vi "Main.vi"() -> ()   [LabVIEW 2016]
doc: "This template is for the Queued Message Handler design pattern.\n\nThe Event Handling Loop generates messages based on user interface actions.\n\nThe Message Handling Loop processes messages generated by the Event Handling Loop, or by other messages. The messages are string values, so new messages can be added easily to the Message Cases case structure in the Message Handling Loop. Each message cluster can also provide an optional value for Message Data, which is a variant that can be converted to whatever message-specific data is required."
uses:
  controls/UI Data.ctl
  controls/Model_Controller Data.ctl
  controls/LV Version Details.ctl
  support/Message Queue/Enqueue Message (Single).vi
  <vilib>/xml/Load XML File.vi
  <vilib>/Utility/error.llb/Error Cluster From Error Code.vi
  <vilib>/ErrorRing/Error Ring.xnode
  support/Message Queue/Message Queue.lvlib
  support/User Event - Stop/User Event - Stop.lvlib
  <vilib>/xml/NI_XML.lvlib
panel:
  in  "OpenInLV":bool
  in  "LV Version":u16(ring) caption="LabVIEW Version" items=["LabVIEW 2014 SP1 32-bit", "LabVIEW 2016 32-bit", "LabVIEW 2017 SP1 32-bit", "LabVIEW 2019 SP1 f1 32-bit"]
  out "Load Time (ms)":u32
  out "DS":T1(array[cluster])
  out "parse errors":string
  in  "LV Project Viewer":string(tree)
  in  "LVProject File Path":path
  in  "Do Something Else <Replace Me>":bool
  in  "Do Something <Replace Me>":bool
  in  "Exit":bool
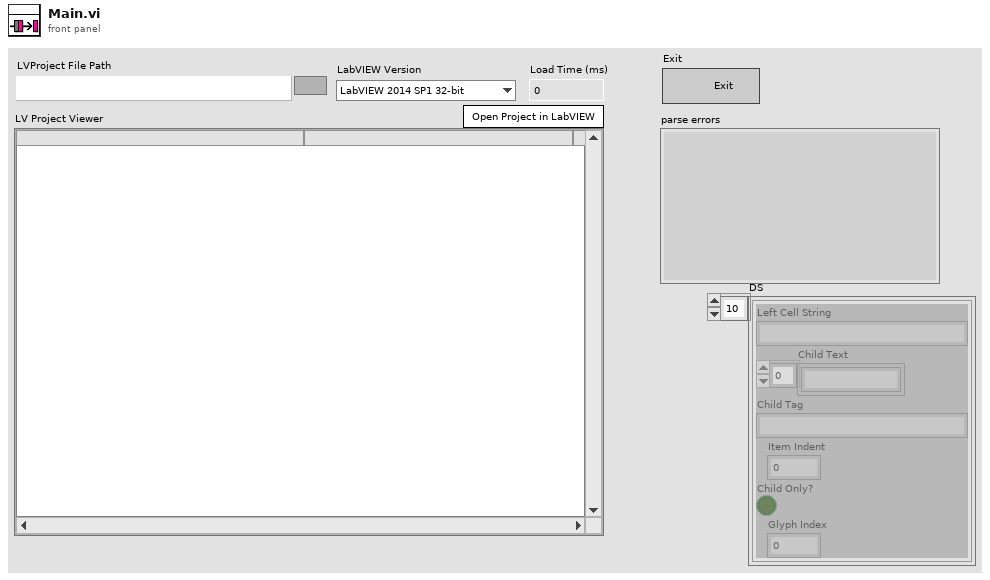
[diagram p1: front panel]
types:
  T1 = cluster{"Left Cell String":string, "Child Text":string[], "Child Tag":string, "Item Indent":i32, "Child Only?":bool, "Glyph Index":i32}[]
  T2 = typedef "Model_Controller Data.ctl" = cluster{"LVProj XML String":string, "LV Proj XML DOM":refnum<k20>, "DS":cluster{"Left Cell String":string, "Child Text":string[], "Child Tag":string, "Item Indent":i32, "Child Only?":bool, "Glyph Index":i32}[], "LV Version Details":T3[], "Selected LV Version":T3, "Item to open in LV":string}
  T3 = typedef "LV Version Details.ctl" = cluster{"Bitness":string, "Version String":string, "LV EXE Path":path, "Display Name":string, "Version":string}
  T4 = typedef "UI Data.ctl" = cluster{"Exit Button Ref":refnum<vi>, "LV Proj File Path":path, "LV Proj View Tree":refnum<vi>}
  T5 = typedef "Message Queue.lvlib/All Message Queues.ctl" = cluster{"UI":refnum<queue>}
  T6 = typedef "imagedata.ctl" = cluster{"image type":i32, "image depth":i32, "image":u8[], "mask":u8[], "colors":u32[], "Rectangle":cluster{"left":i16, "top":i16, "right":i16, "bottom":i16}}
  T7 = cluster{"Left Cell String":string, "Child Text":string[], "Child Tag":string, "Item Indent":i32, "Child Only?":bool, "Glyph Index":i32}
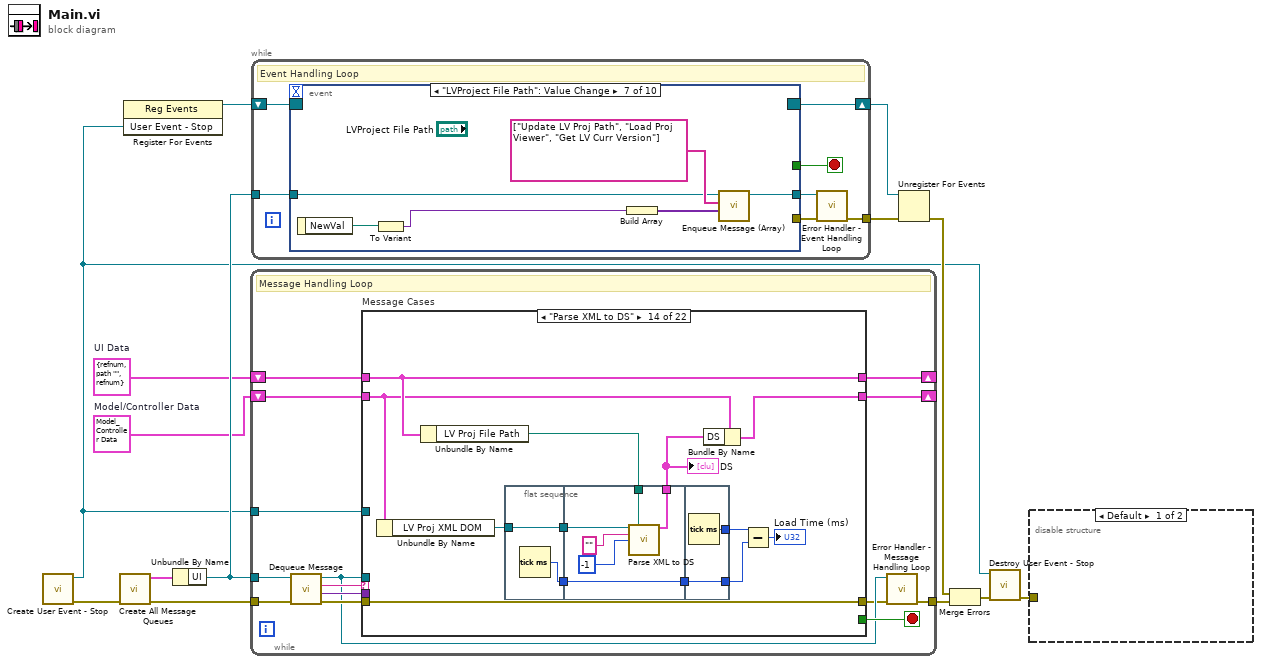
[diagram p0: block diagram]
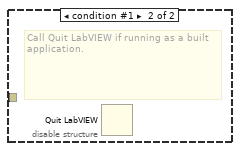
[diagram p2: hidden frame]
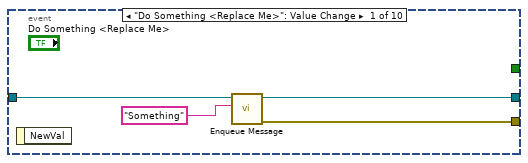
[diagram p3: hidden frame]
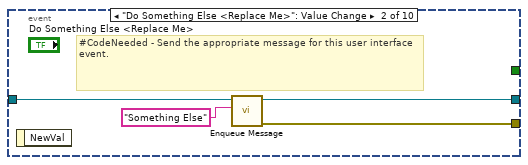
[diagram p4: hidden frame]
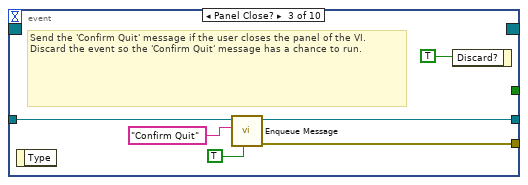
[diagram p5: hidden frame]
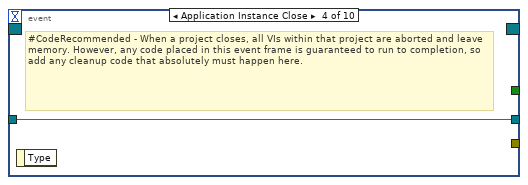
[diagram p6: hidden frame]
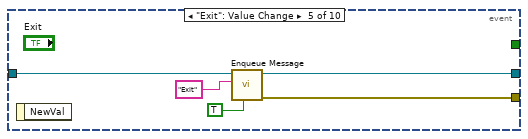
[diagram p7: hidden frame]
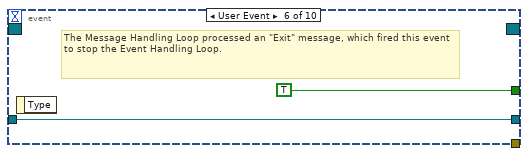
[diagram p8: hidden frame]
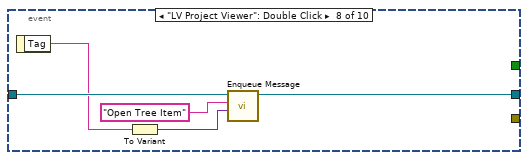
[diagram p9: hidden frame]
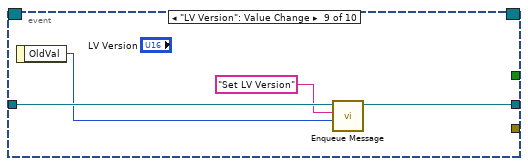
[diagram p10: hidden frame]
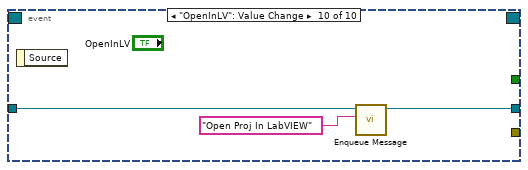
[diagram p11: hidden frame]
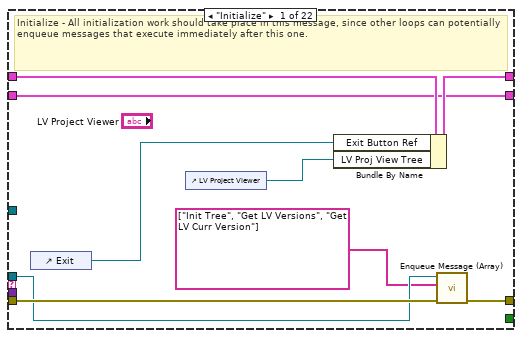
[diagram p12: hidden frame]
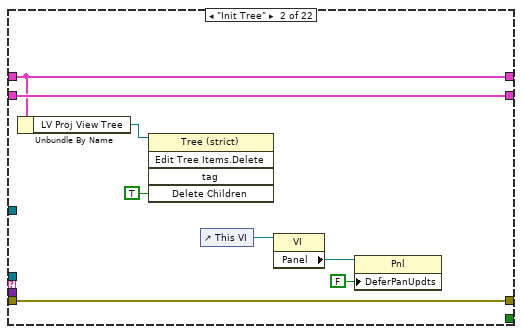
[diagram p13: hidden frame]
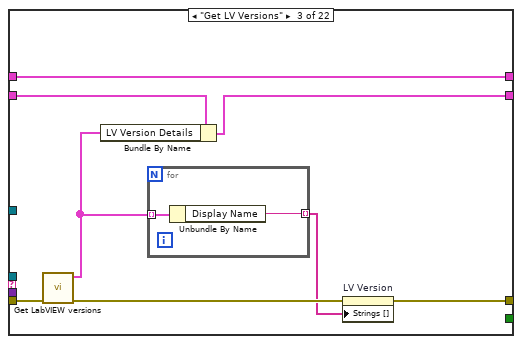
[diagram p14: hidden frame]
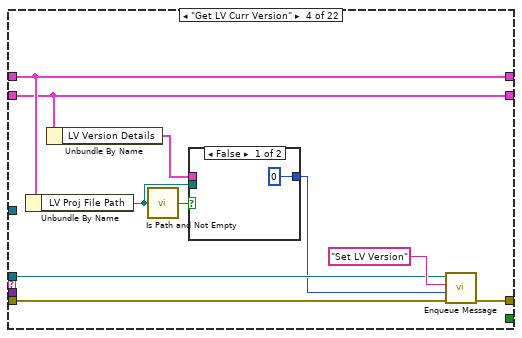
[diagram p15: hidden frame]
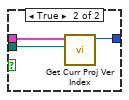
[diagram p16: hidden frame]
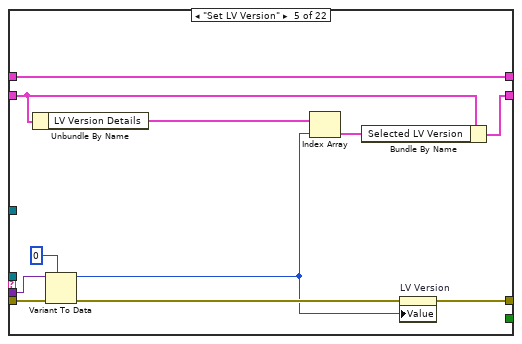
[diagram p17: hidden frame]
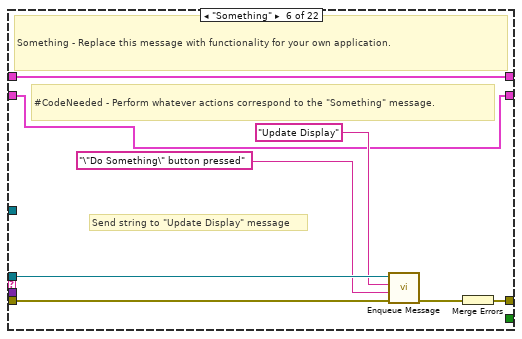
[diagram p18: hidden frame]
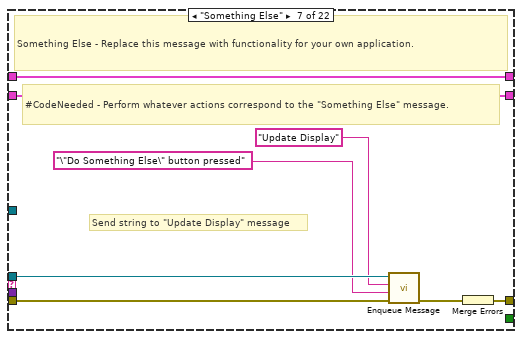
[diagram p19: hidden frame]
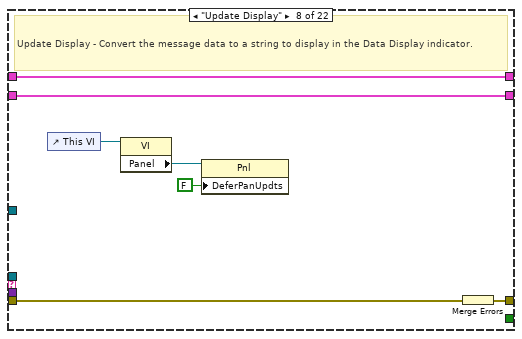
[diagram p20: hidden frame]
diagram:
  w1 = T2 {"LVProj XML String"="", "LV Proj XML DOM"=refnum, "DS"=[], "LV Version Details"=[], "Selected LV Version"={"Bitness"="", "Version String"="", "LV EXE Path"=path "", "Display Name"="", "Version"=""}, "Item to open in LV"=""}  # Model/Controller Data
  w6 = T4 {"Exit Button Ref"=refnum, "LV Proj File Path"=path "", "LV Proj View Tree"=refnum}  # UI Data
  n1 = call "Create User Event - Stop.vi"() -> ("error out"=w10:errorcluster, "User Event - Stop"=w2:refnum<user-event>)  [unwired: 10 in]
  n2 = call "Create All Message Queues.vi"("error in (no error)"=w10) -> ("error out"=w14:errorcluster, "Message Queues out"=w13:T5)  [unwired: 9 in]
  n3 = register-events(w2) -> (reference out=w3:refnum<event-registration>)  [unwired: 2 in, 1 out]
  n4 = Unbundle By Name(w13) -> ("UI"=w11:refnum<queue>)
  n5 = while {
    tunnel: w11 -> [w20]
    shift-right: [w27] -> _
    shift-left: w6 -> [w28]
    tunnel: w2 -> [w25]
    tunnel: w14 -> [w24]
    tunnel: [w18] -> w12
    shift-right: [w15] -> _
    shift-left: w1 -> [w16]
    stop <- w26 stop-if-true
    # "Message Handling Loop"
    n6 = call "Dequeue Message.vi"("error in (no error)"=w24, "Message Queue"=w20) -> ("error out"=w23:errorcluster, "Message Data"=w21:variant, "Message"=w22:string, "dup Message Queue"=w19:refnum<queue>)  [unwired: 6 in]
    n7 = case "Message Cases" shown="\"Parse XML to DS\"" w22 {
      selector: w22 -> [_ _ _ _ _ _ _ _ _ _ _ _ _ _ _ _ _ _ _ _ _ w242]
      tunnel: w19 -> [w30 _ _ w57 _ w84 w92 _ _ w115 w121 _ _ _ _ _ _ w194 w215 _ w240 _]
      tunnel: w23 -> [w32 w45 w52 w59 w79 w86 w94 w101 w111 w119 w123 w133 w142 w156 w172 w183 w190 w205 w217 w224 w233 _]
      tunnel: [w31 w45 w48 w58 w73 w87 w95 w102 w105 w117 w125 w135 w141 w156 w172 w183 w190 w195 w216 w223 w236 w243] -> w17
      tunnel: w28 -> [w37 w42 w53 w63 w80 w88 w96 w103 w110 w118 w126 w128 w143 w154 w170 w178 w189 w200 w218 w222 w239 w244]
      tunnel: [w36 w42 w53 w63 w80 w88 w96 w103 w110 w118 w126 w127 w143 w154 w170 w178 w189 w200 w218 w222 w239 w244] -> w27
      tunnel: [_ _ _ _ _ _ _ _ _ _ _ _ _ _ _ _ _ _ _ _ TRUE _] -> w26
      tunnel: w21 -> [_ _ _ _ w78 _ _ _ w109 _ _ w131 _ _ _ _ _ w204 _ _ w230 _]
      tunnel: w25 -> [_ _ _ _ _ _ _ _ _ _ _ _ _ _ _ _ _ _ _ _ w235 _]
      tunnel: w16 -> [w34 w44 w51 w61 w71 w81 w89 w100 w104 w112 w124 w134 w138 w152 w171 w176 w188 w193 w213 w221 w229 w241]
      tunnel: [w34 w44 w50 w61 w70 w81 w89 w100 w104 w112 w124 w134 w137 w151 w171 w176 w188 w192 w212 w221 w229 w241] -> w15
      frame "Initialize" {
        # "Initialize - All initialization work should take place in this message, since other loops can potentially enqueue messages that execute immediately after this one."
        n8 = control-ref of="Exit"() -> (w35:refnum<vi>)
        n9 = control-ref of="LV Project Viewer"() -> (w33:refnum<vi>)
        n10 = Bundle By Name(cluster=w37, "Exit Button Ref"=w35, "LV Proj View Tree"=w33) -> (w36:T4)
        n11 = call "Enqueue Message (Array).vi"("error in (no error)"=w32, "Message Array"=string[] ["Init Tree", "Get LV Versions", "Get LV Curr Version"], "Message Queue"=w30) -> ("error out"=w31:errorcluster)  [unwired: 7 in, 1 out]
      }
      frame "Init Tree" {
        n12 = Unbundle By Name(w42) -> ("LV Proj View Tree"=w41:refnum<vi>)
        n13 = invoke class="Tree (strict)" method="Edit Tree Items.Delete"(reference=w41, "Delete Children"=TRUE ("Delete Children?")) -> ()  [unwired: 3 in, 5 out]
        n14 = control-ref of="This VI"() -> (w40:refnum<vi>)
        n15 = property class="VI"(reference=w40) -> ("Panel"=w39:refnum<vi>)  [unwired: 1 in, 2 out]
        n16 = property class="Pnl"(reference=w39, "DeferPanUpdts"=FALSE ("Defer Panel Updates")) -> ()  [unwired: 1 in, 2 out]
      }
      frame "Get LV Versions" {
        n17 = call "Get LabVIEW versions.vi"("error in (no error)"=w52) -> ("error out"=w49:errorcluster, "LV Version Details"=w47:T3[])  [unwired: 9 in]
        n18 = Bundle By Name(cluster=w51, "LV Version Details"=w47) -> (w50:T2)
        n19 = for {
          tunnel: w47 -> [w55] mode=indexing
          tunnel: [w54] -> w46 mode=indexing
          n20 = Unbundle By Name(w55) -> ("Display Name"=w54:string)
        }
        n21 = property on="LV Version" class="Ring (strict)"(error in=w49, "Strings []"=w46) -> (error out=w48:errorcluster)  [unwired: 1 in, 1 out]
      }
      frame "Get LV Curr Version" {
        n22 = Unbundle By Name(w63) -> ("LV Proj File Path"=w65:path)
        n23 = Unbundle By Name(w61) -> ("LV Version Details"=w62:T3[])
        n24 = call <vilib>:"Is Path and Not Empty.vi"("path"=w65) -> ("Is Path and Not Empty?"=w64:bool)  [unwired: 4 in]
        n25 = case shown="False" w64 {
          tunnel: w65 -> [_ w69]
          tunnel: w62 -> [_ w68]
          tunnel: [0 ("Proj LV Ver Index") w67] -> w56
          frame False {
          }
          frame True {
            n26 = call "Get Curr Proj Ver Index.vi"("LV Proj File Path"=w69, "LV Version Details"=w68) -> ("Proj LV Ver Index"=w67:i32)  [unwired: 9 in]
          }
        }
        n27 = call-poly "Enqueue Message.vi"("error in (no error)"=w59, "Message Data"=w56, "Message"="Set LV Version", "Message Queue"=w57) -> ("error out"=w58:errorcluster)  [unwired: 6 in, 1 out]
      }
      frame "Set LV Version" {
        n28 = Unbundle By Name(w71) -> ("LV Version Details"=w75:T3[])
        n29 = Variant To Data(error in=w79, type=u16 0, Variant=w78) -> (data=w72:u16, error out=w74:errorcluster)
        n30 = Index Array(array=w75, index=w72) -> (element=w76:T3)
        n31 = Bundle By Name(cluster=w71, "Selected LV Version"=w76) -> (w70:T2)
        n32 = property on="LV Version" class="Ring (strict)"(error in=w74, "Value"=w72) -> (error out=w73:errorcluster)  [unwired: 1 in, 1 out]
      }
      frame "Something" {
        # "Send string to \"Update Display\" message"
        # "#CodeNeeded - Perform whatever actions correspond to the \"Something\" message."
        # "Something - Replace this message with functionality for your own application."
        n33 = call-poly "Enqueue Message.vi"("error in (no error)"=w86, "Message Data"="\"Do Something\" button pressed" ("\"Do Something\" button pressed"), "Message"="Update Display", "Message Queue"=w84) -> ("error out"=w85:errorcluster)  [unwired: 6 in, 1 out]
        n34 = Merge Errors(w85) -> (w87:errorcluster)
      }
      frame "Something Else" {
        # "Send string to \"Update Display\" message"
        # "#CodeNeeded - Perform whatever actions correspond to the \"Something Else\" message."
        # "Something Else - Replace this message with functionality for your own application."
        n35 = call-poly "Enqueue Message.vi"("error in (no error)"=w94, "Message Data"="\"Do Something Else\" button pressed" ("\"Do Something Else\" button pressed"), "Message"="Update Display", "Message Queue"=w92) -> ("error out"=w93:errorcluster)  [unwired: 6 in, 1 out]
        n36 = Merge Errors(w93) -> (w95:errorcluster)
      }
      frame "Update Display" {
        # "Update Display - Convert the message data to a string to display in the Data Display indicator."
        n37 = control-ref of="This VI"() -> (w99:refnum<vi>)
        n38 = property class="VI"(reference=w99) -> ("Panel"=w98:refnum<vi>)  [unwired: 1 in, 2 out]
        n39 = property class="Pnl"(reference=w98, "DeferPanUpdts"=FALSE ("Defer Panel Updates")) -> ()  [unwired: 1 in, 2 out]
        n40 = Merge Errors(w101) -> (w102:errorcluster)
      }
      frame "Error" {
        # "#CodeRecommended - If you ever change the name of this \"Error\" message, you'll need to update the name in the Check Loop Error.vi as well."
        # "#CodeRecommended - Consider creating a system for logging errors in some way. These errors are for notification purposes only. Handling of specific errors should be performed in the message frames that generated the error."
        # "Error - Display an error dialog. This message is sent by the \"Error Handler\" VIs at the end of other loops in this application."
        n41 = Variant To Data(error in=w111, type=errorcluster {"status"=FALSE, "code"=0, "source"=""} ("error constant"), Variant=w109) -> (data=w107:errorcluster, error out=w106:errorcluster)
        n42 = call <vilib>:"Simple Error Handler.vi"("error in (no error)"=w107) -> ()  [unwired: 4 in, 5 out]
        n43 = Merge Errors(w106) -> (w105:errorcluster)
      }
      frame "Confirm Quit" {
        # "#CodeNeeded - If you want to provide an \"Are you sure\" dialog (or some other notification) before the application exits, place that code here. This message is typically sent from a Panel Close? event."
        # "Confirm Quit - Message that can confirm whether or not the user wants to exit the application."
        n44 = call-poly "Enqueue Message.vi"("Priority Message? (F)"=TRUE, "error in (no error)"=w119, "Message"="Exit", "Message Queue"=w115) -> ("error out"=w116:errorcluster)  [unwired: 6 in, 1 out]
        n45 = Merge Errors(w116) -> (w117:errorcluster)
      }
      frame "Load Proj Viewer" {
        n46 = call "Enqueue Message (Array).vi"("error in (no error)"=w123, "Message Array"=string[] ["Init Tree", "Read Proj XML", "Parse XML to DS", "Add Custom Symbols", "Populate Nodes", "Close All", "Update Display"], "Message Queue"=w121) -> ("error out"=w122:errorcluster)  [unwired: 7 in, 1 out]
        n47 = Merge Errors(w122) -> (w125:errorcluster)
      }
      frame "Update LV Proj Path" {
        n48 = Variant To Data(error in=w133, type=path "", Variant=w131) -> (data=w129:path, error out=w132:errorcluster)
        n49 = Bundle By Name(cluster=w128, "LV Proj File Path"=w129) -> (w127:T4)
        n50 = Merge Errors(w132) -> (w135:errorcluster)
      }
      frame "Read Proj XML" {
        n51 = Unbundle By Name(w143) -> ("LV Proj File Path"=w140:path)
        n52 = call-poly <vilib>:"Load.vi"("path to XML document"=w140, "error in (no error)"=w142) -> ("DOM document out"=w139:refnum<k20>, "parse errors"=→"parse errors":string, "error out"=w141:errorcluster)  [unwired: 11 in]
        n53 = Bundle By Name(cluster=w138, "LV Proj XML DOM"=w139) -> (w137:T2)
      }
      frame "Parse XML to DS" {
        n54 = Unbundle By Name(w152) -> ("LV Proj XML DOM"=w155:refnum<k20>)
        n55 = Unbundle By Name(w154) -> ("LV Proj File Path"=w153:path)
        n56 = flat-sequence {
          tunnel: w155 -> [w158]
          tunnel: [w158] -> w150
          tunnel: [w157] -> w146
          tunnel: w153 -> [w161]
          tunnel: [w160] -> w149
          tunnel: w150 -> [w164]
          tunnel: w146 -> [w159]
          tunnel: [w159] -> w145
          tunnel: [w166] -> w147
          tunnel: [w165] -> w144
          tunnel: w145 -> [w165]
          frame #0 {
            n57 = Tick Count (ms)() -> (millisecond timer value=w157:u32)
          }
          frame #1 {
            n58 = call "Parse XML to DS.vi"("Refnum in"=w164, "LV Proj File Path"=w161, "Node Name"="", "Item Indent"=-1) -> ("DS"=w160:T1)  [unwired: 10 in, 1 out]
          }
          frame #2 {
            n59 = Tick Count (ms)() -> (millisecond timer value=w166:u32)
          }
        }
        n60 = Bundle By Name(cluster=w152, "DS"=w149) -> (w151:T2)
        n61 = Subtract(x=w147, y=w144) -> (x-y=→"Load Time (ms)":u32)
        "DS" <- w149
      }
      frame "Add Custom Symbols" {
        n62 = Unbundle By Name(w170) -> ("LV Proj View Tree"=w169:refnum<vi>)
        n63 = call "Glyph Driver.vi"("Op Mode"=enum16{"Get Glyph Index", "Get all Glyphs"}."Get all Glyphs") -> ("FileGlyphs"=w167:T6[])  [unwired: 12 in, 2 out]
        n64 = invoke class="Tree (strict)" method="Custom Item Symbols.Set Symbol Array"(reference=w169, "glyphs"=w167) -> ()  [unwired: 2 in, 4 out]
      }
      frame "Close All" {
        n65 = Unbundle By Name(w176) -> ("DS"=w175:T1)
        n66 = Unbundle By Name(w178) -> ("LV Proj View Tree"=w177:refnum<vi>)
        n67 = Index Array(array=w175) -> (element=w174:T7)  [unwired: 1 in]
        n68 = invoke class="Tree (strict)" method="Open/Close.Open/Close All"(reference=w177, "Open"=FALSE ("Open?")) -> (reference out=w181:refnum<vi>, error out=w180:errorcluster)  [unwired: 2 in, 2 out]
        n69 = Unbundle By Name(w174) -> ("Child Tag"=w173:string)
        n70 = invoke class="Tree (strict)" method="Open/Close.Item"(reference=w181, error in=w180, "tag"=w173, "Open"=TRUE ("Open?")) -> ()  [unwired: 1 in, 5 out]
      }
      frame "Populate Nodes" {
        n71 = Unbundle By Name(w189) -> ("LV Proj View Tree"=w185:refnum<vi>)
        n72 = Unbundle By Name(w188) -> ("DS"=w187:T1)
        n73 = invoke class="Tree (strict)" method="Edit Tree Items.Delete"(reference=w185, "Delete Children"=TRUE ("Delete Children?")) -> (reference out=w184:refnum<vi>)  [unwired: 3 in, 4 out]
        n74 = invoke class="Tree (strict)" method="Edit Tree Items.Add Multiple Items to End"(reference=w184, "Items"=w187) -> ()  [unwired: 2 in, 4 out]
      }
      frame "Open Tree Item" {
        n75 = Unbundle By Name(w193) -> ("DS"=w202:T1)
        n76 = Variant To Data(error in=w205, type="", Variant=w204) -> (data=w201:string, error out=w196:errorcluster)
        n77 = for {
          tunnel: w202 -> [w206] mode=indexing
          tunnel: w201 -> [w208]
          tunnel: [w206] -> w199
          stop <- w207 stop-if-true
          n78 = Unbundle By Name(w206) -> ("Child Tag"=w209:string)
          n79 = Equal?(x=w209, y=w208) -> (x = y?=w207:bool)
        }
        n80 = Unbundle By Name(w199) -> ("Child Text"=w198:string[])
        n81 = Index Array(array=w198) -> (element=w191:string)  [unwired: 1 in]
        n82 = Bundle By Name(cluster=w193, "Item to open in LV"=w191) -> (w192:T2)
        n83 = call-poly "Enqueue Message.vi"("error in (no error)"=w196, "Message"="Open In LabVIEW", "Message Queue"=w194) -> ("error out"=w195:errorcluster)  [unwired: 7 in, 1 out]
      }
      frame "Open Proj In LabVIEW" {
        n84 = Unbundle By Name(w218) -> ("LV Proj File Path"=w211:path)
        n85 = Path To String(path=w211) -> (string=w210:string)
        n86 = Bundle By Name(cluster=w213, "Item to open in LV"=w210) -> (w212:T2)
        n87 = call-poly "Enqueue Message.vi"("error in (no error)"=w217, "Message"="Open In LabVIEW", "Message Queue"=w215) -> ("error out"=w216:errorcluster)  [unwired: 7 in, 1 out]
      }
      frame "Open In LabVIEW" {
        n88 = Unbundle By Name(w221) -> ("Item to open in LV"=w220:string, "Selected LV Version.LV EXE Path"=w219:path)
        n89 = Format Into String(format string="cmd /c labview.exe \"%s\"", w220) -> (resulting string=w227:string)  [unwired: 2 in, 1 out]
        n90 = call <vilib>:"System Exec.vi"("run minimized? (F)"=TRUE, "wait until completion? (T)"=FALSE, "error in (no error)"=w224, "working directory"=w219, "command line"=w227) -> ("error out"=w223:errorcluster)  [unwired: 3 in, 3 out]
      }
      frame "Exit" {
        # "Stop the VI"
        # "Release the message queue reference"
        # "#CodeNeeded - Add any required cleanup code here. Note that if 'Exit' was called as a result of an error, an error dialog will be displayed. Add any custom error handling for an 'Exit' condition here as well."
        # "Exit - Exit the application."
        n91 = Variant To Data(type=errorcluster {"status"=FALSE, "code"=0, "source"=""} ("error constant"), Variant=w230) -> (data=w231:errorcluster)  [unwired: 1 in, 1 out]
        n92 = call <vilib>:"Simple Error Handler.vi"("error in (no error)"=w231) -> ()  [unwired: 4 in, 5 out]
        n93 = call "Fire User Event - Stop.vi"("User Event - Stop"=w235) -> ("error out"=w234:errorcluster)  [unwired: 10 in]
        n94 = Release Queue(queue=w240, error in (no error)=w233) -> (error out=w237:errorcluster)  [unwired: 1 in, 2 out]
        n95 = Merge Errors(w234, w237) -> (w236:errorcluster)
      }
      frame Default {
        # "'Default' case only runs if there is a message that isn't defined in any of the other cases.  Output a programming error."
        n96 = xnode "Error Ring"("parameter 0"=w242) -> ("error out"=w243:errorcluster)
      }
    }
    n97 = call "Error Handler - Message Handling Loop.vi"("error in (no error)"=w17, "Message Queue"=w19) -> ("dup error in"=w18:errorcluster)  [unwired: 8 in, 1 out]
  }
  n98 = while {
    tunnel: w11 -> [w258]
    shift-right: [w256] -> w7
    shift-left: w3 -> [w257]
    tunnel: [w252] -> w4
    stop <- w254 stop-if-true
    # "Event Handling Loop"
    n99 = event shown="[6] \"LVProject File Path\": Value Change" {
      selector: w257 -> [_ _ _ _ _ _ _ _ _ _]
      dyn-events: [_ _ _ _ _ _ _ _ _ _] -> w256
      timeout: _ -> [_ _ _ _ _ _ _ _ _ _]
      tunnel: [_ _ _ _ _ TRUE ("Discard?") _ _ _ _] -> w254
      tunnel: w258 -> [w262 w266 w271 w273 w278 w280 w283 w291 w295 w298]
      tunnel: [w259 w263 w270 _ w277 _ _ _ _ _] -> w255
      tunnel: [w261 w265 w269 w273 w276 w280 w285 w290 w294 w297] -> w253
      event "Do Something <Replace Me>": Value Change {
        n100 = event-data() -> ()  [unwired: 1 in, 1 out]
        n101 = call-poly "Enqueue Message.vi"("Message"="Something", "Message Queue"=w262) -> ("error out"=w259:errorcluster, "dup Message Queue"=w261:refnum<queue>)  [unwired: 8 in]
      }
      event "Do Something Else <Replace Me>": Value Change {
        # "#CodeNeeded - Send the appropriate message for this user interface event."
        n102 = event-data() -> ()  [unwired: 1 in, 1 out]
        n103 = call-poly "Enqueue Message.vi"("Message"="Something Else", "Message Queue"=w266) -> ("error out"=w263:errorcluster, "dup Message Queue"=w265:refnum<queue>)  [unwired: 8 in]
      }
      event Panel Close? {
        # "Send the 'Confirm Quit' message if the user closes the panel of the VI. Discard the event so the 'Confirm Quit' message has a chance to run."
        n104 = event-data() -> ()  [unwired: 1 in, 1 out]
        n105 = call-poly "Enqueue Message.vi"("Priority Message? (F)"=TRUE, "Message"="Confirm Quit", "Message Queue"=w271) -> ("error out"=w270:errorcluster, "dup Message Queue"=w269:refnum<queue>)  [unwired: 7 in]
        n106 = event-data("Discard?"=TRUE) -> ()  [unwired: 1 in, 1 out]
      }
      event Application Instance Close {
        # "#CodeRecommended - When a project closes, all VIs within that project are aborted and leave memory. However, any code placed in this event frame is guaranteed to run to completion, so add any cleanup code that absolutely must happen here."
        n107 = event-data() -> ()  [unwired: 1 in, 1 out]
      }
      event "Exit": Value Change {
        n108 = event-data() -> ()  [unwired: 1 in, 1 out]
        n109 = call-poly "Enqueue Message.vi"("Priority Message? (F)"=TRUE, "Message"="Exit", "Message Queue"=w278) -> ("error out"=w277:errorcluster, "dup Message Queue"=w276:refnum<queue>)  [unwired: 7 in]
      }
      event User Event {
        # "The Message Handling Loop processed an \"Exit\" message, which fired this event to stop the Event Handling Loop."
        n110 = event-data() -> ()  [unwired: 1 in, 1 out]
      }
      event "LVProject File Path": Value Change {
        n111 = event-data() -> ("NewVal"=w286:path)  [unwired: 1 in]
        n112 = To Variant(anything=w286) -> (Variant=w282:variant)
        n113 = Build Array(w282) -> (w281:variant[])
        n114 = call "Enqueue Message (Array).vi"("Message Data Array"=w281, "Message Array"=string[] ["Update LV Proj Path", "Load Proj Viewer", "Get LV Curr Version"], "Message Queue"=w283) -> ("dup Message Queue"=w285:refnum<queue>)  [unwired: 7 in, 1 out]
      }
      event "LV Project Viewer": Double Click {
        n115 = event-data() -> ("Tag"=w288:string)  [unwired: 1 in]
        n116 = To Variant(anything=w288) -> (Variant=w287:variant)
        n117 = call-poly "Enqueue Message.vi"("Message Data"=w287, "Message"="Open Tree Item", "Message Queue"=w291) -> ("dup Message Queue"=w290:refnum<queue>)  [unwired: 7 in, 1 out]
      }
      event "LV Version": Value Change {
        n118 = event-data() -> ("OldVal"=w292:u16)  [unwired: 1 in]
        n119 = call-poly "Enqueue Message.vi"("Message Data"=w292, "Message"="Set LV Version", "Message Queue"=w295) -> ("dup Message Queue"=w294:refnum<queue>)  [unwired: 7 in, 1 out]
      }
      event "OpenInLV": Value Change {
        n120 = event-data() -> ()  [unwired: 1 in, 1 out]
        n121 = call-poly "Enqueue Message.vi"("Message"="Open Proj In LabVIEW", "Message Queue"=w298) -> ("dup Message Queue"=w297:refnum<queue>)  [unwired: 8 in, 1 out]
      }
    }
    n122 = call "Error Handler - Event Handling Loop.vi"("error in (no error)"=w255, "Message Queue"=w253) -> ("dup error in"=w252:errorcluster)  [unwired: 8 in, 1 out]
  }
  n123 = Unregister For Events(event registration refnum=w7, error in=w4) -> (error out=w8:errorcluster)
  n124 = Merge Errors(w8, w12) -> (w9:errorcluster)
  n125 = call "Destroy User Event - Stop.vi"("error in (no error)"=w9, "User Event - Stop"=w2) -> ("error out"=w5:errorcluster)  [unwired: 9 in]
  n126 = disable-structure shown="Default" {
    disable-tunnel: w5 -> [_ _]
    frame condition #0 (active) {
    }
    frame condition #1 {
      # "Call Quit LabVIEW if running as a built application."
      n127 = Quit LabVIEW() -> ()  [unwired: 1 in]
    }
  }
